vi "RichToFlatrfcontrol_DeviceRequest.vi"(5 "OutputClusterType":T1, 11 "InputCluster":T2) -> (3 "OutputCluster":T1)   [LabVIEW 2024, in "FlexSDR_gRPC_client.lvlib"]
uses:
  FlexSDR_gRPC_client.lvlib
  rfcontrol_DeviceRequest.ctl
  rfcontrol_DeviceRequest_Flat.ctl
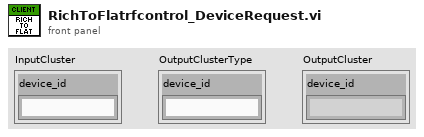
[diagram p1: front panel]
types:
  T1 = typedef "FlexSDR_gRPC_client.lvlib/rfcontrol_DeviceRequest_Flat.ctl" = cluster{"device_id":string}
  T2 = typedef "FlexSDR_gRPC_client.lvlib/rfcontrol_DeviceRequest.ctl" = cluster{"device_id":string}
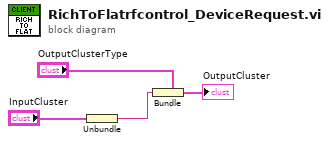
[diagram p0: block diagram]
diagram:
  n1 = Unbundle "Unbundle"("InputCluster") -> ("device_id"=w1:string)
  n2 = Bundle "Bundle"(cluster="OutputClusterType", "device_id"=w1) -> (→"OutputCluster":T1)
